vi "Auto 1.vi"() -> ()   [LabVIEW 2018]
uses:
  2019 Swerve Test Chassis/SwerveChassis2019Test 2.3/Robot Global Data.vi
panel:
  in  "Encoders":T1
  in  "PID Gains":T2={"X PID"={"proportional gain (Kc)"=0.02000000000000001, "integral time (Ti, min)"=0.0, "derivative time (Td, min)"=0.0}, "Y PID"={"proportional gain (Kc)"=0.02000000000000001, "integral time (Ti, min)"=0.0, "derivative time (Td, min)"=0.0}, "Z PID"={"proportional gain (Kc)"=0.02000000000000001, "integral time (Ti, min)"=0.0, "derivative time (Td, min)"=0.0}} {"Z PID"."derivative time (Td, min)" format="%.3f"; "Z PID"."integral time (Ti, min)" format="%.3f"; "Z PID"."proportional gain (Kc)" format="%.3f"; "Y PID"."derivative time (Td, min)" format="%.3f"; "Y PID"."integral time (Ti, min)" format="%.3f"; "Y PID"."proportional gain (Kc)" format="%.3f"; "X PID"."derivative time (Td, min)" format="%.3f"; "X PID"."integral time (Ti, min)" format="%.3f"; "X PID"."proportional gain (Kc)" format="%.3f"}
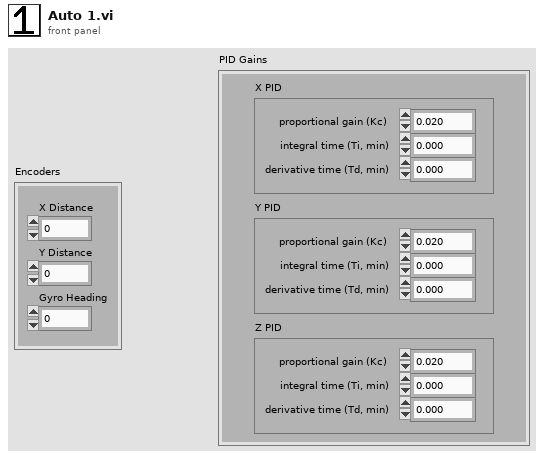
[diagram p1: front panel]
types:
  T1 = cluster{"X Distance":dbl, "Y Distance":dbl, "Gyro Heading":dbl}
  T2 = cluster{"X PID":cluster{"proportional gain (Kc)":dbl, "integral time (Ti, min)":dbl, "derivative time (Td, min)":dbl}, "Y PID":cluster{"proportional gain (Kc)":dbl, "integral time (Ti, min)":dbl, "derivative time (Td, min)":dbl}, "Z PID":cluster{"proportional gain (Kc)":dbl, "integral time (Ti, min)":dbl, "derivative time (Td, min)":dbl}}
  T3 = cluster{"X Dist.":dbl, "Y Dist.":dbl, "Gyro":dbl}
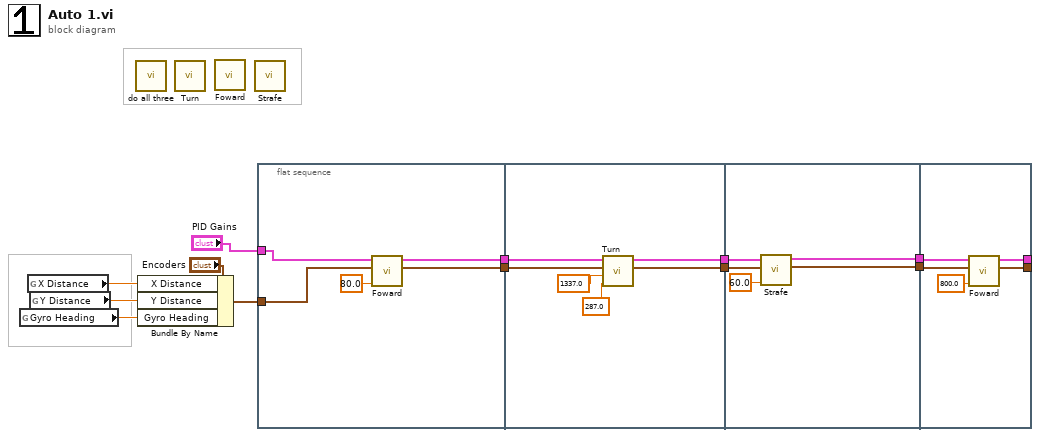
[diagram p0: block diagram]
diagram:
  n1 = global read "Robot Global Data.vi" "Gyro Heading"() -> (w12:dbl)
  n2 = global read "Robot Global Data.vi" "X Distance"() -> (w10:dbl)
  n3 = global read "Robot Global Data.vi" "Y Distance"() -> (w11:dbl)
  n4 = call "do all three.vi"() -> ()  [unwired: 12 in]
  n5 = Bundle By Name(cluster="Encoders", "X Distance"=w10, "Y Distance"=w11, "Gyro Heading"=w12) -> (w8:T1)
  n6 = call "Turn.vi"() -> ()  [unwired: 10 in, 2 out]
  n7 = call "Foward.vi"() -> ()  [unwired: 9 in, 2 out]
  n8 = call "Strafe.vi"() -> ()  [unwired: 10 in, 2 out]
  n9 = flat-sequence {
    tunnel: w8 -> [w16]
    tunnel: "PID Gains" -> [w17]
    tunnel: [w15] -> w6
    tunnel: [w14] -> w5
    tunnel: w6 -> [w23]
    tunnel: w5 -> [w22]
    tunnel: [w21] -> w4
    tunnel: [w20] -> w3
    tunnel: w4 -> [w27]
    tunnel: w3 -> [w28]
    tunnel: [w26] -> w2
    tunnel: [w25] -> w1
    tunnel: w2 -> [w33]
    tunnel: w1 -> [w32]
    tunnel: [w31] -> _
    tunnel: [w30] -> _
    frame #0 {
      n10 = call "Foward.vi"("PID Gains In"=w17, "Encoders In"=w16, "Y Target"=80.0) -> ("PID Gains Out"=w15:T2, "Encoders Out"=w14:T3)  [unwired: 6 in]
    }
    frame #1 {
      n11 = call "Turn.vi"("Gyro Target"=287.0, "Y Target"=1337.0, "Encoders In"=w22, "PID Gains In"=w23) -> ("Encoders Out"=w20:T3, "PID Gains Out"=w21:T2)  [unwired: 6 in]
    }
    frame #2 {
      n12 = call "Strafe.vi"("X target"=60.0, "Encoders In"=w28, "PID Gains In"=w27) -> ("Encoders Out"=w25:T3, "PID Gains Out"=w26:T2)  [unwired: 7 in]
    }
    frame #3 {
      n13 = call "Foward.vi"("PID Gains In"=w33, "Encoders In"=w32, "Y Target"=800.0) -> ("PID Gains Out"=w31:T2, "Encoders Out"=w30:T3)  [unwired: 6 in]
    }
  }
